vi "Align Buffers.vi"(8 "error in (no error)":errorcluster, 10 "Plugin Buffers":refnum<class "Buffers.lvclass">, 11 "Transfer Group in":refnum<class "Transfer Group.lvclass">) -> (0 "error out":errorcluster, 3 "Transfer Group out":refnum<class "Transfer Group.lvclass">)   [LabVIEW 2017, in "DSF Core.lvlib" / "Transfer Group.lvclass"]
uses:
  Transfer Group.lvclass
  Buffer/Buffers.lvclass
  Transfer Group.lvclass/Transfer Group.ctl
  Transfer/Transfer.lvclass
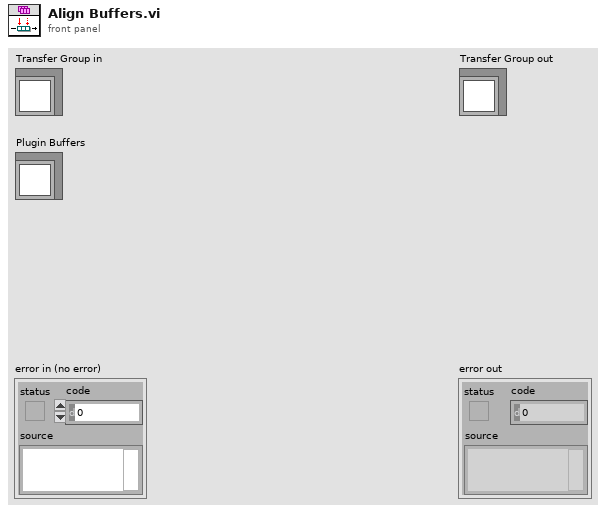
[diagram p1: front panel]
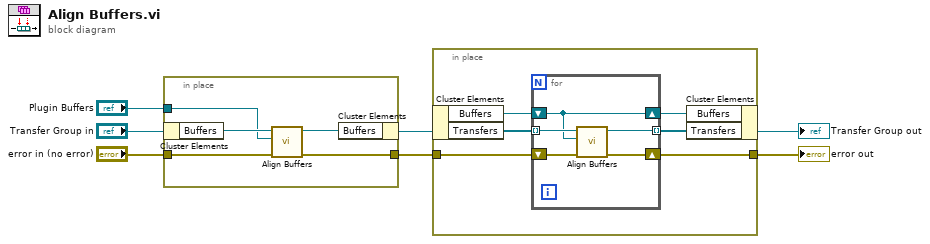
[diagram p0: block diagram]
diagram:
  n1 = in-place {
    in-place-border: "error in (no error)" -> [w11]
    in-place-border: [w10] -> w1
    in-place-border: "Plugin Buffers" -> [w8]
    n2 = in-place-cluster #1("Transfer Group in") -> ("Buffers"=w12:refnum<class "Buffers.lvclass">)
    n3 = call "Align Buffers.vi"("error in (no error)"=w11, "base Buffers"=w8, "Buffers in"=w12) -> ("error out"=w10:errorcluster, "Buffers out"=w9:refnum<class "Buffers.lvclass">)  [unwired: 7 in]
    n4 = in-place-cluster #1("Buffers"=w9) -> (w3:refnum<class "Transfer Group.lvclass">)
  }
  n5 = in-place {
    in-place-border: [w16] -> w7
    in-place-border: w1 -> [w15]
    n6 = in-place-cluster #2(w3) -> ("Buffers"=w14:refnum<class "Buffers.lvclass">, "Transfers"=w18:refnum<class "Transfer.lvclass">[])
    n7 = for {
      tunnel: w18 -> [w23] mode=indexing
      tunnel: [w21] -> w17 mode=indexing
      shift-right: [w20] -> w16
      shift-left: w15 -> [w22]
      shift-right: [w19] -> w13
      shift-left: w14 -> [w19]
      n8 = call "Align Buffers.vi"("error in (no error)"=w22, "Transfer Group Buffers"=w19, "Transfer in"=w23) -> ("error out"=w20:errorcluster, "Transfer out"=w21:refnum<class "Transfer.lvclass">)  [unwired: 7 in]
    }
    n9 = in-place-cluster #2("Buffers"=w13, "Transfers"=w17) -> (→"Transfer Group out":refnum<class "Transfer Group.lvclass">)
  }
  "error out" <- w7
